vi "Read Leaf.vi"(11 "TEMPLATE Actor in":refnum<class "TEMPLATE Actor.lvclass">) -> (2 "Leaf":bool)   [LabVIEW 2020, in "_Template.lvlib" / "Templates.lvlib" / "TEMPLATE jettl Actor.lvlib" / "TEMPLATE Actor.lvlib" / "TEMPLATE Actor.lvclass"]
uses:
  TEMPLATE Actor.lvclass
  TEMPLATE Actor.lvclass/TEMPLATE Actor.ctl
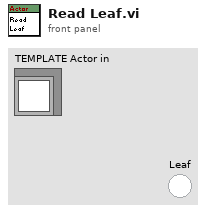
[diagram p1: front panel]
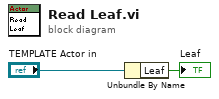
[diagram p0: block diagram]
diagram:
  n1 = Unbundle By Name("TEMPLATE Actor in") -> ("Leaf"=→"Leaf":bool)
